vi "NodeAdjust.vi"(1 "PicAjust":T1={"TranslationVector"=[], "scale"=1.0, "Pitch（x) "=0.0, "Yaw（y)"=0.0, "Roll（z) "=0.0} {"Roll（z)" scale=-90.0..90.0; "Yaw（y)" scale=-90.0..90.0; "Pitch（x)" scale=-90.0..90.0}, 2 "NodeM":dbl[][](array[numeric])=[[50.0, 50.0, 500.0], [500.0, 50.0, 500.0], [500.0, 350.0, 500.0], [50.0, 350.0, 500.0], [50.0, 50.0, 500.0]], 3 "视图":enum16{"俯视图", "轴测图"}(ring)) -> (0 "NewNodeM":dbl[][](array[numeric]))   [LabVIEW 2014]
doc: "数据通过四元数法调整节点"
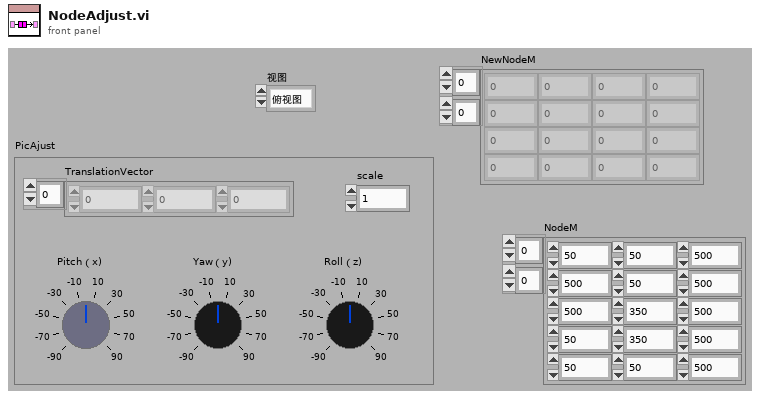
[diagram p1: front panel]
types:
  T1 = cluster{"TranslationVector":dbl[], "scale":dbl, "Pitch（x) ":dbl, "Yaw（y)":dbl, "Roll（z) ":dbl}
  T2 = typedef "NI_Kinematics.lvlib/Quaternion.ctl" = dbl[]
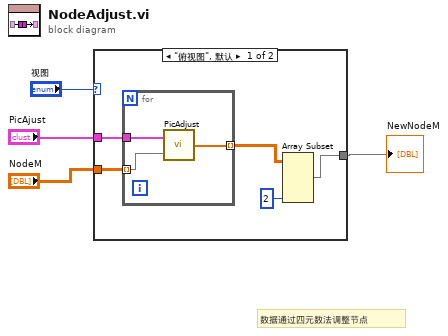
[diagram p0: block diagram]
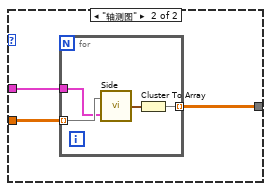
[diagram p2: hidden frame]
diagram:
  # "数据通过四元数法调整节点"
  n1 = case shown="\"俯视图\", 默认" "视图" {
    tunnel: "NodeM" -> [w8 w15]
    tunnel: "PicAjust" -> [w9 w14]
    tunnel: [w5 w13] -> w1
    frame "俯视图", Default {
      n2 = for {
        tunnel: w9 -> [w12]
        tunnel: w8 -> [w11] mode=indexing
        tunnel: [w10] -> w7 mode=indexing
        n3 = call "PicAdjust.vi"("Input"=w11, "PicAjust"=w12) -> ("子数组"=w10:T2)
      }
      n4 = Array Subset(array=w7, length (col)=2 ("长度")) -> (w5:dbl[][])  [unwired: 3 in]
    }
    frame "轴测图" {
      n5 = for {
        tunnel: w15 -> [w19] mode=indexing
        tunnel: w14 -> [w18]
        tunnel: [w17] -> w13 mode=indexing
        n6 = call "Side.vi"("PicAjust"=w18, "Input"=w19) -> ("输出簇"=w16:cluster{"x":dbl, "y":dbl})
        n7 = Cluster To Array(cluster=w16) -> (array=w17:dbl[])
      }
    }
  }
  "NewNodeM" <- w1
